vi "Write.vi"(8 "error in (no error)":errorcluster, 10 "data":string, 11 "pipe writer in":refnum<data-value>) -> (0 "error out":errorcluster, 1 "bytes written":i32, 3 "pipe writer out":refnum<data-value>)   [LabVIEW 2013, in "Linux RT IPC.lvlib" / "Pipes.lvlib" / "Unix Pipe Writer.lvclass"]
doc: "This VI writes a certain number of bytes to the provided pipe endpoint."
uses:
  Unix Pipe Writer.lvclass
  Unix Pipe/Unix Pipe.lvclass/Unix Pipe.ctl
  Unix Pipe/Unix Pipe.lvclass
  C/C.lvlib
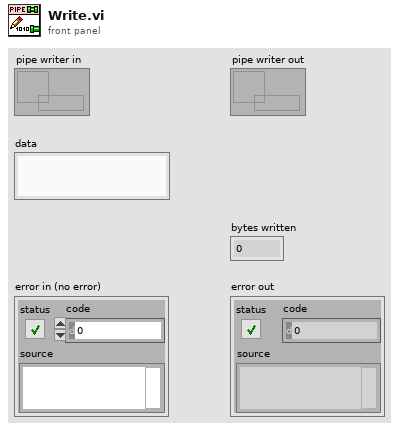
[diagram p1: front panel]
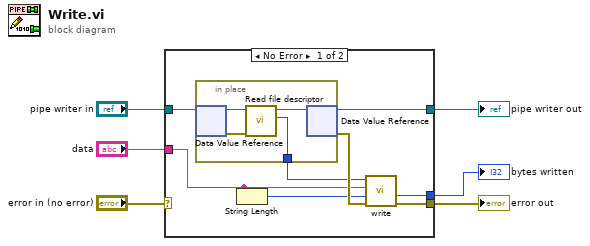
[diagram p0: block diagram]
diagram:
  n1 = case shown="No Error" "error in (no error)" {
    selector: "error in (no error)" -> [_ w19]
    tunnel: "pipe writer in" -> [w14 w20]
    tunnel: [w13 w20] -> w4
    tunnel: [w11 w19] -> w3
    tunnel: [w9 _] -> w2
    tunnel: "data" -> [w8 _]
    frame No Error {
      n2 = in-place {
        in-place-border: [w16] -> w10
        n3 = in-place-dvr #1(w14) -> (w18:refnum<class "Unix Pipe Writer.lvclass">, w17:errorcluster)
        n4 = call "Read file descriptor.vi"("error in (no error)"=w17, "Unix Pipe in"=w18) -> ("file descriptor"=w16:i32, "Unix Pipe out"=w15:refnum<class "Unix Pipe Writer.lvclass">)  [unwired: 7 in, 1 out]
        n5 = in-place-dvr #1(w15) -> (w13:refnum<data-value>, w12:errorcluster)
      }
      n6 = String Length(string=w8) -> (length=w7:i32)
      n7 = call "write.vi"("error in (no error)"=w12, "bytes to write"=w7, "data"=w8, "file descriptor in"=w10) -> ("error out"=w11:errorcluster, "bytes written"=w9:i32)  [unwired: 5 in, 1 out]
    }
    frame Error {
    }
  }
  "error out" <- w3
  "pipe writer out" <- w4
  "bytes written" <- w2
